vi "Get 1D Array String.vi"(5 "use temporary file? (F)":bool, 7 "data type of variable":string[](array[string]), 8 "error in":errorcluster, 10 "variable name":string, 11 "GOLPI ref. in":T1={"pipe handle"={"lv_proc.dll file path"=path "", "process instance handle"=[]}, "fast read timeout [ms]"=500, "fast read settle time [ms]"=10, "fast read to multiple [ms]"=1, "max elements per input line"=100, "slow read timeout [ms]"=5000, "stdin double format specifier"="%_16e", "max elements per stdout output column"=100}) -> (0 "error out":errorcluster, 2 "value":string[](array[string]), 3 "GOLPI ref. out":T1={"pipe handle"={"lv_proc.dll file path"=path "", "process instance handle"=[]}, "fast read timeout [ms]"=500, "fast read settle time [ms]"=10, "fast read to multiple [ms]"=1, "max elements per input line"=100, "slow read timeout [ms]"=5000, "stdin double format specifier"="%_16e", "max elements per stdout output column"=100})   [LabVIEW 2013, in "GOLPI library.lvlib"]
doc: "Part of polymorph Get Variable.vi"
uses:
  GOLPI library.lvlib
  Type Definitions/GOLPI reference Type Def.ctl
  LV Process source distribution/Pipe Handle.ctl
  Type Definitions/Custom Error Codes Enum Type Def.vi
  LV Process source distribution/LV Process library.lvlib
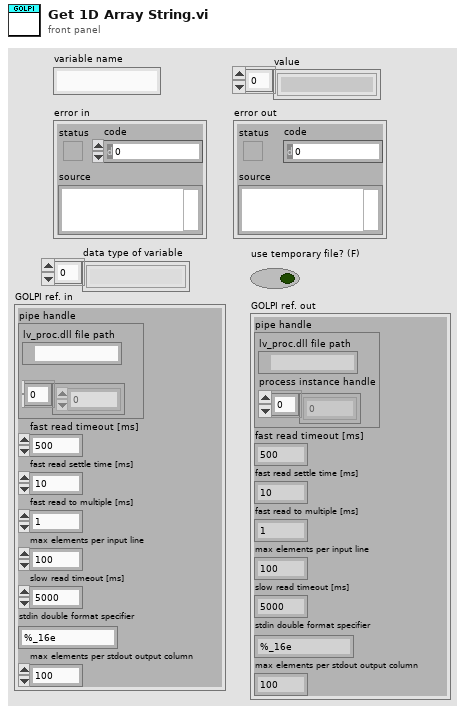
[diagram p1: front panel]
types:
  T1 = typedef "GOLPI library.lvlib/GOLPI reference Type Def.ctl" = cluster{"pipe handle":T2, "fast read timeout [ms]":u32, "fast read settle time [ms]":u32, "fast read to multiple [ms]":u32, "max elements per input line":u32, "slow read timeout [ms]":u32, "stdin double format specifier":string, "max elements per stdout output column":u32}
  T2 = typedef "LV Process library.lvlib/Pipe Handle.ctl" = cluster{"lv_proc.dll file path":path, "process instance handle":u32[]}
  T3 = typedef "GOLPI library.lvlib/Custom Error Codes Enum Type Def.vi" = enum16{"no error", "00 working directory PAR1 missing", "01 octave binary PAR1 missing", "02 octave report error PAR1", "03 empty output last cmd PAR1", "04 missing temporary file PAR1", "05 pwd PAR 1 not exist", "10 var PAR1 not string, vect", "11 var PAR1 not num, scal, ~compl", "12 var PAR1 not num, scal, compl", "13 var PAR1 not num, vect, ~compl", "14 var PAR1 not num, vect, compl", "15 var PAR1 not num, mat, ~compl", "16 var PAR1 not num, mat, ~compl", "30 WARNING read timeout", "99 not finished"}
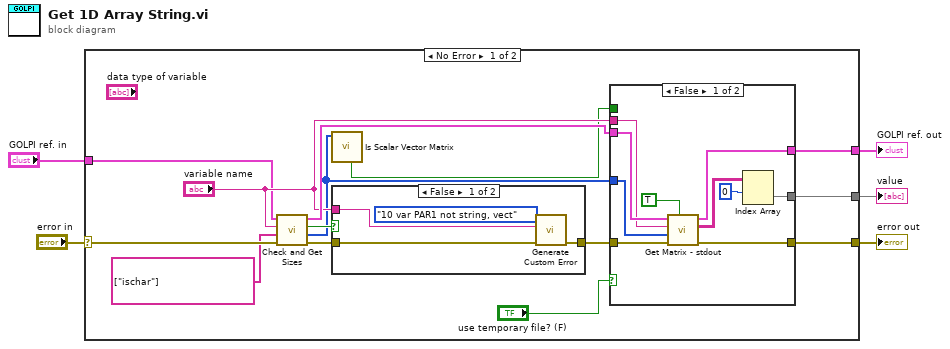
[diagram p0: block diagram]
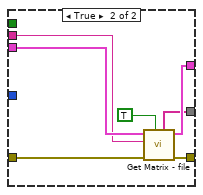
[diagram p2: hidden frame]
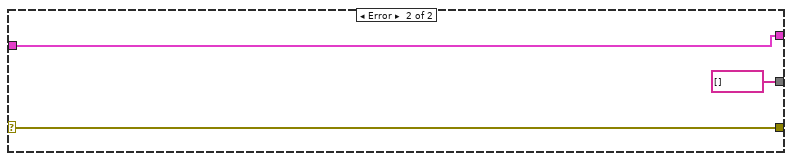
[diagram p4: hidden frame]
diagram:
  n1 = case shown="No Error" "error in" {
    selector: "error in" -> [w17 w44]
    tunnel: [w12 w44] -> w5
    tunnel: [w19 string[] [] ("vector")] -> w3
    tunnel: "GOLPI ref. in" -> [w9 w42]
    tunnel: [w8 w42] -> w1
    frame No Error {
      n2 = call "Check and Get Sizes.vi"("error in (no error)"=w17, "test commands"=string[] ["ischar"], "variable name"="variable name", "GOLPI ref. in"=w9) -> ("error out"=w16:errorcluster, "octave sizes"=w7:i32[], "all tests OK?"=w18:bool, "GOLPI ref. out"=w14:T1)  [unwired: 4 in]
      n3 = call "Is Scalar Vector Matrix.vi"("octave sizes"=w7) -> ("row vector?"=w6:bool)  [unwired: 5 in, 5 out]
      n4 = case shown="False" w18 {
        tunnel: w16 -> [w40 w41]
        tunnel: [w37 w41] -> w13
        tunnel: "variable name" -> [w38 _]
        frame False {
          n5 = call "Generate Custom Error.vi"("error in"=w40, "PAR1"=w38, "GOLPI error"=Custom_Error_Codes_Enum_Type_Def.vi."10 var PAR1 not string, vect" ("Enum")) -> ("error out"=w37:errorcluster)  [unwired: 8 in]
        }
        frame True {
        }
      }
      n6 = case shown="False" "use temporary file? (F)" {
        tunnel: [w20 w31] -> w19
        tunnel: w14 -> [w29 w34]
        tunnel: w7 -> [w22 _]
        tunnel: w13 -> [w28 w36]
        tunnel: [w27 w35] -> w12
        tunnel: "variable name" -> [w21 w32]
        tunnel: [w26 w33] -> w8
        tunnel: w6 -> [_ _]
        frame False {
          n7 = call "Get Matrix - stdout.vi"("is string?"=TRUE ("is string"), "error in (no error)"=w28, "octave sizes"=w22, "variable name"=w21, "GOLPI ref. in"=w29) -> ("error out"=w27:errorcluster, "array"=w23:string[][], "GOLPI ref. out"=w26:T1)  [unwired: 4 in]
          n8 = Index Array(array=w23, index (row)=0) -> (element=w20:string[])  [unwired: 1 in]
        }
        frame True {
          n9 = call "Get Matrix - file.vi"("is string?"=TRUE ("is string"), "error in (no error)"=w36, "variable name"=w32, "GOLPI ref. in"=w34) -> ("error out"=w35:errorcluster, "GOLPI ref. out"=w33:T1, "string array"=w31:string[])  [unwired: 3 in, 2 out]
        }
      }
    }
    frame Error {
    }
  }
  "value" <- w3
  "error out" <- w5
  "GOLPI ref. out" <- w1
